vi "Stop Core.vi"(10 "final error code":i32 caption="code d'erreur final", 11 "Cooler in":refnum<class "Cooler.lvclass"> caption="Acteur en entrée") -> (3 "Cooler out":refnum<class "Cooler.lvclass"> caption="Acteur en sortie")   [LabVIEW 2015, in "Cooler.lvlib" / "Cooler.lvclass"]
doc: "(<B>Nom de fichier</B> : Actor Framework.lvlib:Actor.lvclass:Stop Core.vi)\n\nDéfinit ce que l'acteur fait avant de s'arrêter. Utilisez l'entrée <B>code d'erreur final</B> pour déterminer si l'acteur se ferme en réponse à une erreur.\n\nPar défaut, cette méthode ne fait rien. Une classe descendante peut la redéfinir pour configurer un comportement, tel que la fermeture des processus initialisés par l'acteur dans sa redéfinition de la méthode Noyau d'acteur."
uses:
  Cooler.lvclass
  Cooler.lvclass/Cooler.ctl
  <vilib>/ActorFramework/Stop Msg/Stop Msg.lvclass/Stop Msg.ctl
  <vilib>/ActorFramework/Message Enqueuer/Message Enqueuer.lvclass/Message Enqueuer.ctl
  <vilib>/ActorFramework/Stop Msg/Send Emergency Stop.vi
  <vilib>/ActorFramework/Stop Msg/Send Normal Stop.vi
  <vilib>/ActorFramework/Message Enqueuer/Enqueue Critical.vi
  <vilib>/ActorFramework/Message Enqueuer/Enqueue.vi
  <vilib>/ActorFramework/Message Priority Queue/Priority Enqueue.vi
  <vilib>/ActorFramework/Stop Msg/Stop Msg.lvclass
  Level Controller/Level Controller/Level Controller.lvclass
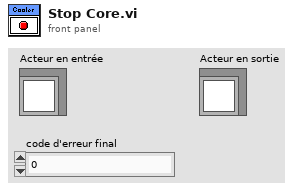
[diagram p1: front panel]
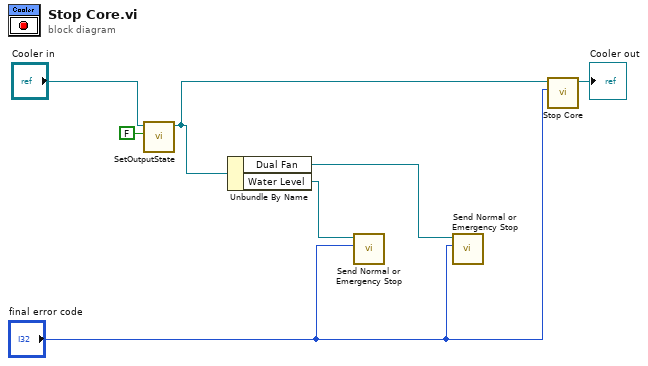
[diagram p0: block diagram]
diagram:
  n1 = call-dynamic "SetOutputState.vi"("Output State"=FALSE, "Cooler in"="Cooler in") -> ("Cooler out"=w4:refnum<class "Cooler.lvclass">)  [unwired: 8 in, 1 out]
  n2 = Unbundle By Name(w4) -> ("Dual Fan"=w3:refnum<class "Message Enqueuer.lvclass">, "Water Level"=w2:refnum<class "Message Enqueuer.lvclass">)
  n3 = call <vilib>:"Send Normal or Emergency Stop.vi"("final error code"="final error code", "Message Enqueuer"=w2) -> ()  [unwired: 9 in, 1 out]
  n4 = call <vilib>:"Send Normal or Emergency Stop.vi"("final error code"="final error code", "Message Enqueuer"=w3) -> ()  [unwired: 9 in, 1 out]
  n5 = call-parent "Stop Core.vi"("final error code"="final error code", "Actor in"=w4) -> ("Actor out"=→"Cooler out":refnum<class "Cooler.lvclass">)  [unwired: 9 in]
